vi "Tarf Angle Updater.vi"(8 "mult":dbl, 10 "AIDeviceRef":T1) -> ()   [LabVIEW 2012]
uses:
  <vilib>/Rock Robotics/WPI/AnalogChannel/WPI_AnalogChannelDevRef.ctl
  <vilib>/Rock Robotics/SystemInterfaces/Typedef/FPGA_TypedefAnalogModule.ctl
  <vilib>/Rock Robotics/SystemInterfaces/AI/FPGA_AIChannel.ctl
  Robot Global Data.vi
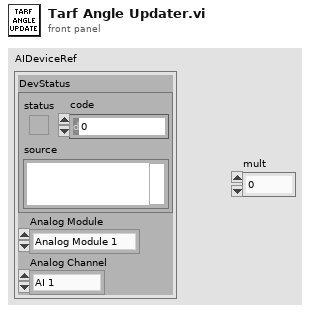
[diagram p1: front panel]
types:
  T1 = typedef "WPI_AnalogChannelDevRef.ctl" = cluster{"DevStatus":errorcluster, "Analog Module":T2, "Analog Channel":T3}
  T2 = typedef "FPGA_TypedefAnalogModule.ctl" = enum16{"Analog Module 1", "Analog Module 2"}
  T3 = typedef "FPGA_AIChannel.ctl" = enum8{"AI 1", "AI 2", "AI 3", "AI 4", "AI 5", "AI 6", "AI 7", "AI 8", "Invalid"}
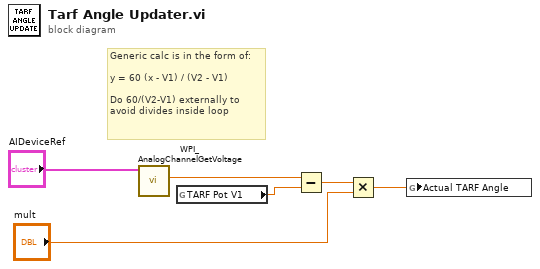
[diagram p0: block diagram]
diagram:
  # "Generic calc is in the form of:\n\ny = 60 (x - V1) / (V2 - V1)\n\nDo 60/(V2-V1) externally to\navoid divides inside loop"
  n1 = call <vilib>:"WPI_AnalogChannelGetVoltage.vi"("AIDeviceRef"="AIDeviceRef") -> ("Voltage"=w5:dbl)  [unwired: 8 in, 2 out]
  n2 = global read "Robot Global Data.vi" "TARF Pot V1"() -> (w4:dbl)
  n3 = Subtract(x=w5, y=w4) -> (x-y=w3:dbl)
  n4 = Multiply(x=w3, y="mult") -> (x*y=w1:dbl)
  n5 = global write "Robot Global Data.vi" "Actual TARF Angle"(w1) -> ()
